vi "Test Criteria Global.vi"() -> ()   [LabVIEW 2013]
uses:
  Pass Weighting.ctl
panel:
  in  "Override Blocking Signal Level (dBm)":dbl=30.0
  in  "Speed Throttle":bool
  out "Required Vdd":dbl format="%#_g V"
  out "Required Temperature":dbl format="%#_g°C"
  out "UUT Vdd":dbl=3.0 format="%#_g V"
  out "UUT Tempreature":dbl=25.0 format="%#_g°C"
  in  "Result Emulation":T1
  in  "Carrier (MHz)":u32=2426
  in  "Packets to Transmit":u32=1500
  in  "PER Pass Rate":dbl=30.8 min=0.0 max=100.0
  # "Emulation Parameters"
  # "Test System Variables"
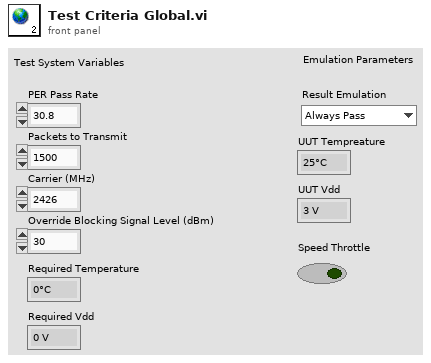
[diagram p1: front panel]
types:
  T1 = typedef "Pass Weighting.ctl" = enum16{"Always Pass", "Always Fail", "Always 30%", "Always 31%", "Random"}
diagram:
